vi "Save-Load AOL Properties.vi"(8 "error in":errorcluster, 9 "AOL Properties IN":T1={"AOD 1 thickness (mm)"=118.0, "AOD 2 thickness (mm)"=115.0, "AOD 3 thickness (mm)"=110.0, "AOD 4 thickness (mm)"=135.0, "AOD 5 thickness (mm)"=135.0, "AOD 6 thickness (mm)"=135.0, "AOD 1-2 separation (mm)"=15.0, "AOD 2-3 separation (mm)"=15.0, "AOD 3-4 separation (mm)"=15.0, "AOD 4-5 separation (mm)"=15.0, "AOD 5-6 separation (mm)"=15.0, "AOD 1 X Offset"=15.0, "AOD 2 X Offset"=1.0, "AOD 3 X Offset"=1.0, "AOD 4 X Offset"=1.0, "AOD 1 Y Offset"=1.0, "AOD 2 Y Offset"=1.0, "AOD 3 Y Offset"=1.0, "AOD 4 Y Offset"=1.0, "AOD 1 X Direction"=0.0, "AOD 2 X Direction"=0.0, "AOD 3 X Direction"=0.0, "AOD 4 X Direction"=0.0, "AOD 1 Y Direction"=1.0, "AOD 2 Y Direction"=0.0, "AOD 3 Y Direction"=0.0023, "AOD 4 Y Direction"=0.0046, "AOD 1 Centre (mm)"=15.0, "AOD 2 Centre (mm)"=50.0, "AOD 3 Centre (mm)"=50.0, "AOD 4 Centre (mm)"=50.0, "Timing Offset AOD 1"=0.0, "Timing Offset AOD 2"=0.0, "Timing Offset AOD 3"=0.0, "Timing Offset AOD 4"=0.0, "AOD Optical offset 1"=20000.0, "AOD Optical offset 2"=20000.0, "AOL aperture (mm)"=15.0, "AOL centre wavelength (nm)"=1.0, "AOL centre frequency (MHz)"=1.0, "Diffraction mode"=1.0, "Crystal length (mm)"=0.0, "Acoustic velocity (m/s)"=1.0, "Pair deflection ratio"=1.0, "AOD fill time (us)"=1.0, "AOD Ord. Refractive index"=2.22, "AOD ExtraOrd. Refractive index"=2.22}, 11 "Function":T2=enum."Load from file") -> (0 "error out":errorcluster, 1 "AOL Properties OUT":T1={"AOD 1 thickness (mm)"=118.0, "AOD 2 thickness (mm)"=115.0, "AOD 3 thickness (mm)"=110.0, "AOD 4 thickness (mm)"=135.0, "AOD 5 thickness (mm)"=135.0, "AOD 6 thickness (mm)"=135.0, "AOD 1-2 separation (mm)"=15.0, "AOD 2-3 separation (mm)"=15.0, "AOD 3-4 separation (mm)"=15.0, "AOD 4-5 separation (mm)"=15.0, "AOD 5-6 separation (mm)"=15.0, "AOD 1 X Offset"=15.0, "AOD 2 X Offset"=1.0, "AOD 3 X Offset"=1.0, "AOD 4 X Offset"=1.0, "AOD 1 Y Offset"=1.0, "AOD 2 Y Offset"=1.0, "AOD 3 Y Offset"=1.0, "AOD 4 Y Offset"=1.0, "AOD 1 X Direction"=0.0, "AOD 2 X Direction"=0.0, "AOD 3 X Direction"=0.0, "AOD 4 X Direction"=0.0, "AOD 1 Y Direction"=1.0, "AOD 2 Y Direction"=0.0, "AOD 3 Y Direction"=0.0023, "AOD 4 Y Direction"=0.0046, "AOD 1 Centre (mm)"=15.0, "AOD 2 Centre (mm)"=50.0, "AOD 3 Centre (mm)"=50.0, "AOD 4 Centre (mm)"=50.0, "Timing Offset AOD 1"=0.0, "Timing Offset AOD 2"=0.0, "Timing Offset AOD 3"=0.0, "Timing Offset AOD 4"=0.0, "AOD Optical offset 1"=20000.0, "AOD Optical offset 2"=20000.0, "AOL aperture (mm)"=15.0, "AOL centre wavelength (nm)"=1.0, "AOL centre frequency (MHz)"=1.0, "Diffraction mode"=1.0, "Crystal length (mm)"=0.0, "Acoustic velocity (m/s)"=1.0, "Pair deflection ratio"=1.0, "AOD fill time (us)"=1.0, "AOD Ord. Refractive index"=2.22, "AOD ExtraOrd. Refractive index"=2.22})   [LabVIEW 2017]
uses:
  Typedefs/AOL Properties Cluster.ctl
  Typedefs/Save-Load enum.ctl
  Typedefs/Which path.ctl
  <vilib>/Utility/config.llb/NI_LVConfig.lvlib
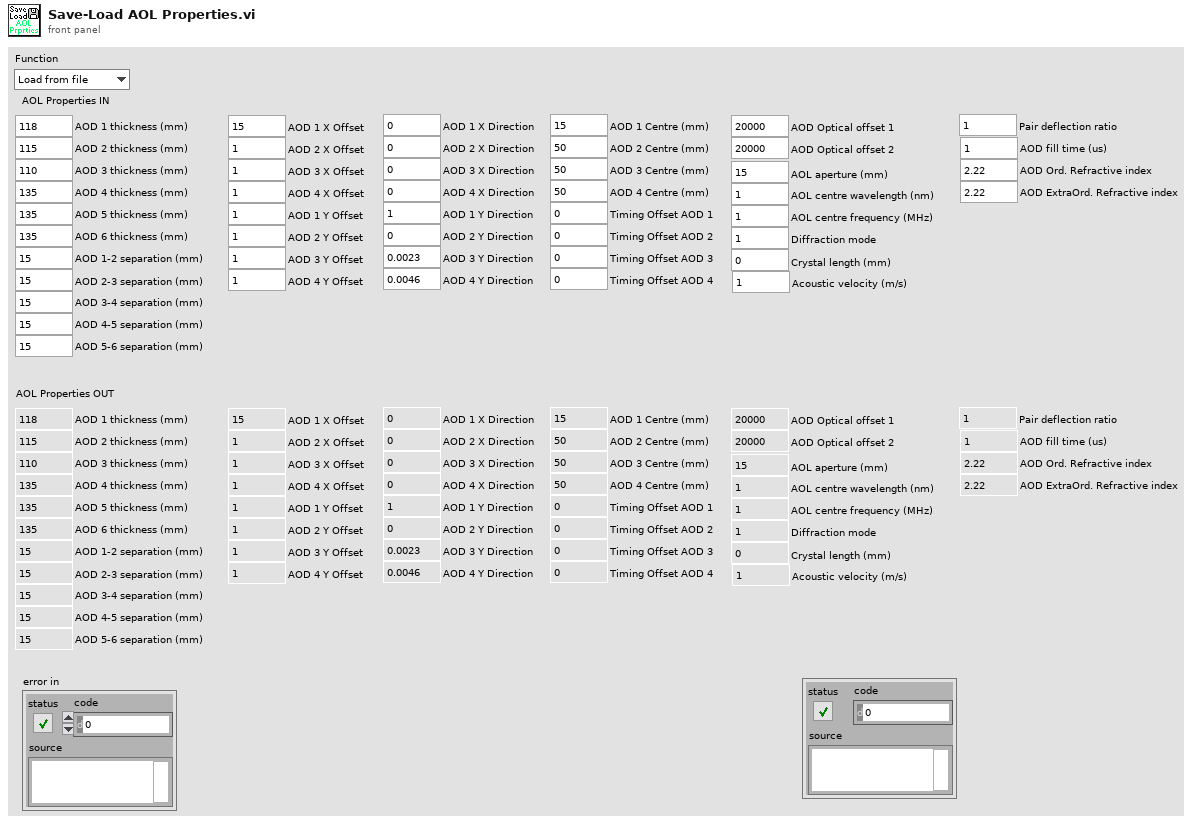
[diagram p1: front panel]
types:
  T1 = typedef "AOL Properties Cluster.ctl" = cluster{"AOD 1 thickness (mm)":dbl, "AOD 2 thickness (mm)":dbl, "AOD 3 thickness (mm)":dbl, "AOD 4 thickness (mm)":dbl, "AOD 5 thickness (mm)":dbl, "AOD 6 thickness (mm)":dbl, "AOD 1-2 separation (mm)":dbl, "AOD 2-3 separation (mm)":dbl, "AOD 3-4 separation (mm)":dbl, "AOD 4-5 separation (mm)":dbl, "AOD 5-6 separation (mm)":dbl, "AOD 1 X Offset":dbl, "AOD 2 X Offset":dbl, "AOD 3 X Offset":dbl, "AOD 4 X Offset":dbl, "AOD 1 Y Offset":dbl, "AOD 2 Y Offset":dbl, "AOD 3 Y Offset":dbl, "AOD 4 Y Offset":dbl, "AOD 1 X Direction":dbl, "AOD 2 X Direction":dbl, "AOD 3 X Direction":dbl, "AOD 4 X Direction":dbl, "AOD 1 Y Direction":dbl, "AOD 2 Y Direction":dbl, "AOD 3 Y Direction":dbl, "AOD 4 Y Direction":dbl, "AOD 1 Centre (mm)":dbl, "AOD 2 Centre (mm)":dbl, "AOD 3 Centre (mm)":dbl, "AOD 4 Centre (mm)":dbl, "Timing Offset AOD 1":dbl, "Timing Offset AOD 2":dbl, "Timing Offset AOD 3":dbl, "Timing Offset AOD 4":dbl, "AOD Optical offset 1":dbl, "AOD Optical offset 2":dbl, "AOL aperture (mm)":dbl, "AOL centre wavelength (nm)":dbl, "AOL centre frequency (MHz)":dbl, "Diffraction mode":dbl, "Crystal length (mm)":dbl, "Acoustic velocity (m/s)":dbl, "Pair deflection ratio":dbl, "AOD fill time (us)":dbl, "AOD Ord. Refractive index":dbl, "AOD ExtraOrd. Refractive index":dbl}
  T2 = typedef "Save-Load enum.ctl" = enum16{"Save to file", "Load from file", "Compare from file"}
  T3 = typedef "Which path.ctl" = enum16{"Configuration Files", "Calibration Files", "Images", "Setup.ini", "Loaded User profile.ini", "User's-Previous session.ini", "New user profile.ini", "Selected User profile.ini", "User profiles folder", "Power meter scaling.txt", "FOV Cal.ini", "Calibration.ini"}
  T4 = typedef "NI_LVConfig.lvlib/Config Data RefNum.ctl" = refnum<k1>
  T5 = typedef "Ini file interface (DBL).ctl" = cluster{"key":string, "Save?":bool, "Default":dbl}[]
  T6 = typedef "Ini file interface (String).ctl" = cluster{"key":string, "Save?":bool, "Default":string}[]
  T7 = typedef "Ini file interface (Boolean).ctl" = cluster{"key":string, "Save?":bool, "Default":bool}[]
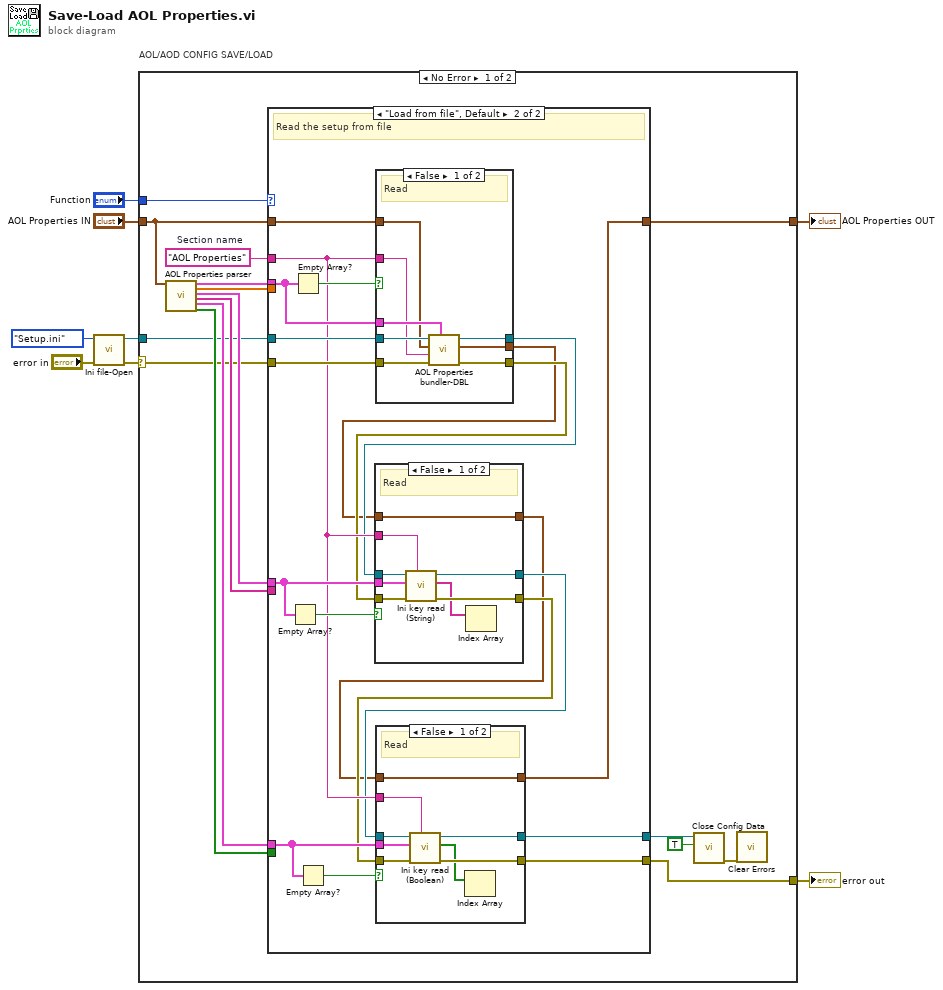
[diagram p0: block diagram]
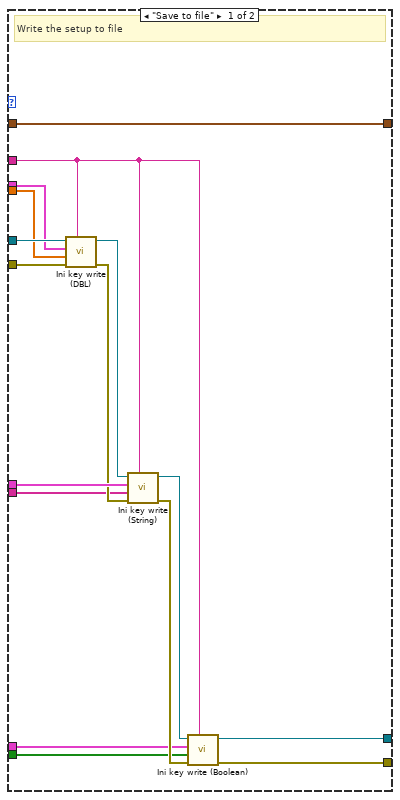
[diagram p2: hidden frame]
diagram:
  n1 = call "Ini file-Open.vi"("Error In"="error in", "Which file?"=Which_path."Setup.ini") -> ("error out"=w4:errorcluster, "User profile ini file ref"=w2:T4)  [unwired: 6 in, 2 out]
  n2 = case "AOL/AOD CONFIG SAVE/LOAD" shown="No Error" w4 {
    selector: w4 -> [w11 w94]
    tunnel: [w9 w94] -> w1
    tunnel: "AOL Properties IN" -> [w19 w93]
    tunnel: [w20 w93] -> w7
    tunnel: "Function" -> [w12 _]
    tunnel: w2 -> [w10 _]
    frame No Error {
      w24 = "AOL Properties"  # Section name
      n3 = call "AOL Properties parser.vi"("AOL Properties"=w19) -> ("Keys setup.DBL"=w18:T5, "Values.DBL"=w17:dbl[], "Keys setup.String"=w16:T6, "Values.Strings"=w15:string[], "Keys setup.Boolean"=w14:T7, "Values.Boolean"=w13:bool[])  [unwired: 13 in]
      n4 = case shown="\"Load from file\", Default" w12 {
        tunnel: [w27 w54] -> w9
        tunnel: [w26 w55] -> w22
        tunnel: w11 -> [w39 w56]
        tunnel: w10 -> [w40 w59]
        tunnel: w24 -> [w29 w49]
        tunnel: w18 -> [w37 w58]
        tunnel: w17 -> [w38 _]
        tunnel: w13 -> [w28 _]
        tunnel: w14 -> [w30 w53]
        tunnel: w15 -> [w33 _]
        tunnel: w16 -> [w36 w50]
        tunnel: [w25 w41] -> w20
        tunnel: w19 -> [w25 w44]
        frame "Save to file" {
          # "Write the setup to file"
          n5 = call "Ini key write (DBL).vi"("Section"=w29, "error in (no error)"=w39, "Values (DBL)"=w38, "Ini file interface"=w37, "Ini file refnum in"=w40) -> ("error out"=w34:errorcluster, "Ini file refnum out"=w35:T4)  [unwired: 5 in]
          n6 = call "Ini key write (String).vi"("Section"=w29, "error in (no error)"=w34, "Values (String)"=w33, "Ini file interface"=w36, "Ini file refnum in"=w35) -> ("error out"=w31:errorcluster, "Ini file refnum out"=w32:T4)  [unwired: 5 in]
          n7 = call "Ini key write (Boolean).vi"("Section"=w29, "error in (no error)"=w31, "Values (Boolean)"=w28, "Ini file interface"=w30, "Ini file refnum in"=w32) -> ("error out"=w27:errorcluster, "Ini file refnum out"=w26:T4)  [unwired: 5 in]
        }
        frame "Load from file", Default {
          # "Read the setup from file"
          n8 = Empty Array?(array=w50) -> (empty?=w51:bool)
          n9 = Empty Array?(array=w58) -> (empty?=w57:bool)
          n10 = Empty Array?(array=w53) -> (empty?=w52:bool)
          n11 = case shown="False" w57 {
            tunnel: w59 -> [w89 w92]
            tunnel: [w88 w92] -> w45
            tunnel: [w87 w91] -> w46
            tunnel: w56 -> [w86 w91]
            tunnel: w49 -> [w84 _]
            tunnel: w58 -> [w85 _]
            tunnel: w44 -> [w83 w90]
            tunnel: [w82 w90] -> w43
            frame False {
              # "Read"
              n12 = call "AOL Properties bundler-DBL.vi"("Keys setup.DBL"=w85, "error in (no error)"=w86, "Section name"=w84, "AOL Properties"=w83, "Refnum in"=w89) -> ("error out"=w87:errorcluster, "AOL Properties"=w82:T1, "Refnum out"=w88:T4)  [unwired: 4 in]
            }
            frame True {
              # "No parametersof such type"
            }
          }
          n13 = case shown="False" w51 {
            tunnel: [w64 w70] -> w48
            tunnel: [w63 w69] -> w47
            tunnel: w50 -> [w66 _]
            tunnel: w45 -> [w67 w70]
            tunnel: w46 -> [w62 w69]
            tunnel: w49 -> [w65 _]
            tunnel: w43 -> [w60 w68]
            tunnel: [w60 w68] -> w42
            frame False {
              # "Read"
              n14 = call "Ini key read (String).vi"("Section name"=w65, "error in (no error)"=w62, "Keys setup"=w66, "Ini file ref in"=w67) -> ("error out"=w63:errorcluster, "Value read/used"=w61:string[], "Ini file ref"=w64:T4)  [unwired: 5 in]
              n15 = Index Array(array=w61) -> ()  [unwired: 1 in, 1 out]
            }
            frame True {
              # "No parametersof such type"
            }
          }
          n16 = case shown="False" w52 {
            tunnel: [w77 w81] -> w55
            tunnel: [w76 w80] -> w54
            tunnel: w53 -> [w73 _]
            tunnel: w48 -> [w78 w81]
            tunnel: w47 -> [w75 w80]
            tunnel: w49 -> [w74 _]
            tunnel: w42 -> [w71 w79]
            tunnel: [w71 w79] -> w41
            frame False {
              # "Read"
              n17 = call "Ini key read (Boolean).vi"("Section"=w74, "error in (no error)"=w75, "Parameter names & setup"=w73, "Ini file refnum in"=w78) -> ("error out"=w76:errorcluster, "Value read/used"=w72:bool[], "Ini file refnum out"=w77:T4)  [unwired: 5 in]
              n18 = Index Array(array=w72) -> ()  [unwired: 1 in, 1 out]
            }
            frame True {
              # "No parametersof such type"
            }
          }
        }
      }
      n19 = call <vilib>:"Close Config Data.vi"("write file if changed (T)"=TRUE ("write configuration file? (F)"), "refnum"=w22) -> ("error out"=w21:errorcluster)  [unwired: 8 in, 1 out]
      n20 = call <vilib>:"Clear Errors.vi"("error in (no error)"=w21) -> ()  [unwired: 5 in, 2 out]
    }
    frame Error {
    }
  }
  "error out" <- w1
  "AOL Properties OUT" <- w7
